vi "Read.vi"(6 "Append Index":i32, 8 "error in (no error)":errorcluster, 11 "Data.TDMS":refnum<class "LV-Data.TDMS.lvclass">) -> (0 "error out":errorcluster, 1 "Notes":string, 2 "Data (Dictionary)":T1[](array[typedef]), 3 "Data.TDMS out":refnum<class "LV-Data.TDMS.lvclass">, 5 "Path out":path)   [LabVIEW 2019, in "LV-Data.TDMS.lvclass"]
uses:
  LV-Data.TDMS.lvclass
  C:/Users/patrick/Documents/GitHub/LV-Data/src/LV-Data/LV-Data.lvclass
  LV-Data/Typedefs/Dictionary--cluster.ctl
  LV-Data.TDMS.lvclass/LV-Data.TDMS.ctl
  LV-Data/Typedefs/Operation--enum.ctl
  LV-Data/LV-Data.lvclass/LV-Data.ctl
  LV-Data/LV-Data.lvclass
  LV-Data/Typedefs/Map Variant--map.ctl
  <vilib>/Utility/miscctls.llb/LVMapReplaceAction.ctl
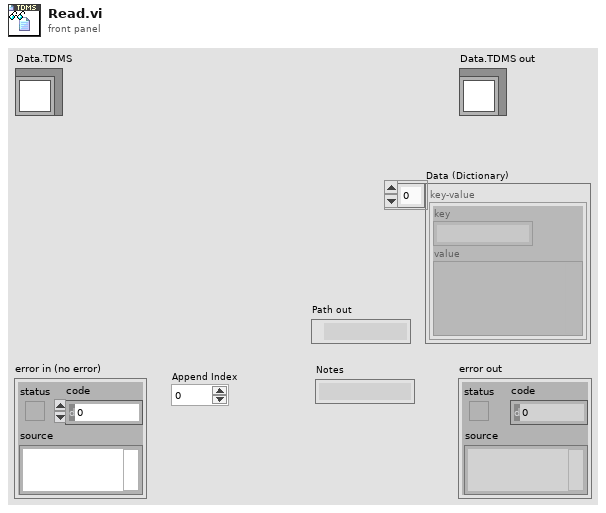
[diagram p1: front panel]
types:
  T1 = typedef "LV-Data.lvclass/Dictionary--cluster.ctl" = cluster{"key":string, "value":variant}
  T2 = typedef "LV-Data.lvclass/Operation--enum.ctl" = enum16{"Read", "Write", "Write + Append"}
  T3 = typedef "LV-Data.lvclass/Map Variant--map.ctl" = map{string, variant}
  T4 = typedef "LVMapReplaceAction.ctl" = enum32{"Modify Entry only if found", "Add or Modify Entry", "Delete Entry"}
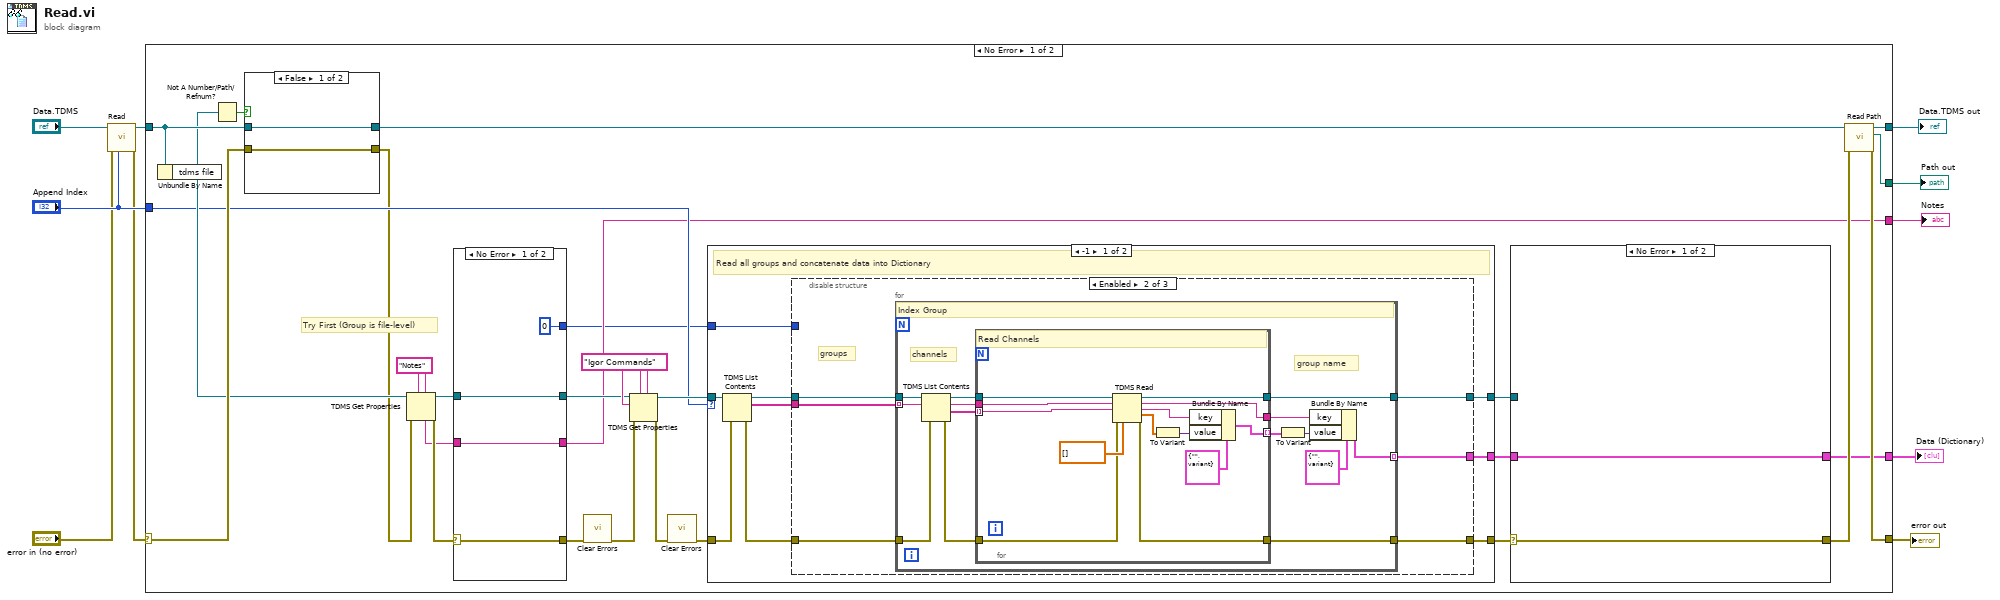
[diagram p0: block diagram]
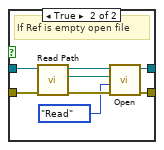
[diagram p2: hidden frame]
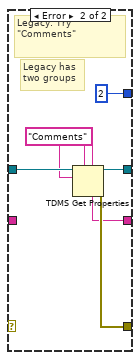
[diagram p3: hidden frame]
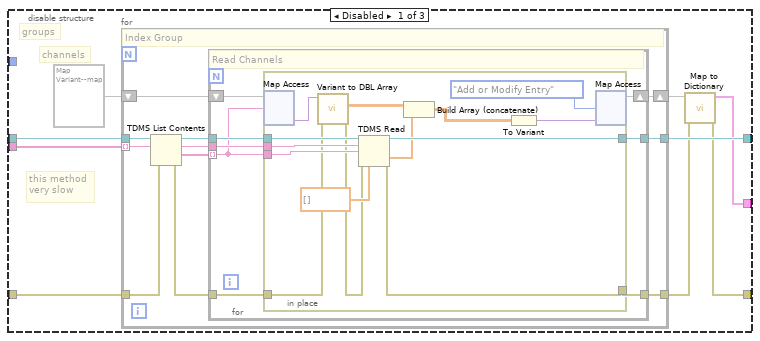
[diagram p4: hidden frame]
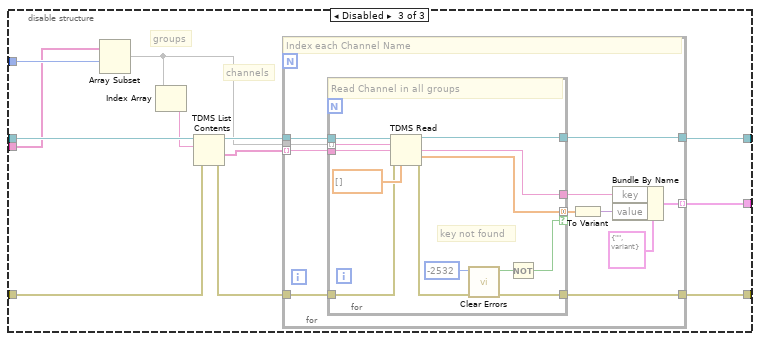
[diagram p5: hidden frame]
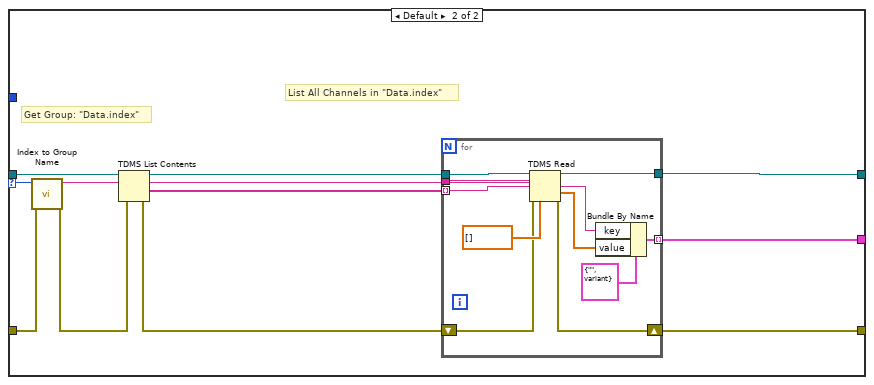
[diagram p6: hidden frame]
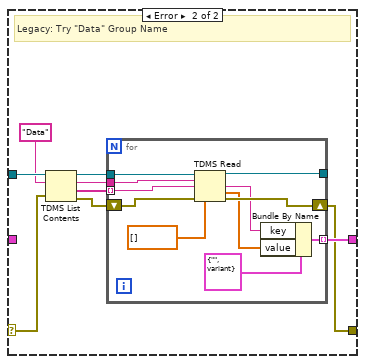
[diagram p7: hidden frame]
diagram:
  n1 = call-parent "Read.vi"("Append Index"="Append Index", "error in (no error)"="error in (no error)", "Data Save in"="Data.TDMS") -> ("error out"=w1:errorcluster, "Data Save out"=w4:refnum<class "LV-Data.TDMS.lvclass">)  [unwired: 4 in, 3 out]
  n2 = case shown="No Error" w1 {
    selector: w1 -> [w31 w223]
    tunnel: w4 -> [w33 w222]
    tunnel: [w36 w222] -> w10
    tunnel: [w35 w223] -> w9
    tunnel: [w37 _] -> w8
    tunnel: "Append Index" -> [w23 _]
    tunnel: [w13 _] -> w7
    tunnel: [w20 _] -> w6
    frame No Error {
      w27 = "Notes" ("group name")
      w30 = "Igor Commands" ("attrib name")
      # "Try First (Group is file-level)"
      n3 = Unbundle By Name(w33) -> ("tdms file"=w25:refnum<k34>)
      n4 = Not A Number/Path/Refnum?(number/path/refnum=w25) -> (NaN/Path/Refnum?=w34:bool)
      n5 = case shown="False" w34 {
        tunnel: w33 -> [w39 w47]
        tunnel: [w39 w48] -> w32
        tunnel: [w40 w44] -> w18
        tunnel: w31 -> [w40 w43]
        frame False {
        }
        frame True {
          # "If Ref is empty open file"
          n6 = call "Read Path.vi"("error in (no error)"=w43, "Data Save"=w47) -> ("error out"=w46:errorcluster, "Path"=w41:path, "Data Save out"=w45:refnum<class "LV-Data.TDMS.lvclass">)  [unwired: 7 in]
          n7 = call-dynamic "Open.vi"("error in (no error)"=w46, "Operation"=Operation--enum."Read", "Path"=w41, "Data.TDMS in"=w45) -> ("error out"=w44:errorcluster, "Data.TDMS out"=w48:refnum<class "LV-Data.TDMS.lvclass">)  [unwired: 6 in]
        }
      }
      n8 = TDMS Get Properties(5:w27, 7:w27, 8:w18, 11:w25) -> (0:w29:errorcluster, 3:w26:refnum<k34>, 4:w28:string)  [unwired: 2 in, 3 out]
      n9 = case shown="No Error" w29 {
        selector: w29 -> [w52 _]
        tunnel: [w52 w58] -> w17
        tunnel: w28 -> [w51 _]
        tunnel: [w51 w57] -> w13
        tunnel: w26 -> [w50 w56]
        tunnel: [w50 w55] -> w24
        tunnel: [0 ("index") 2 ("index")] -> w12
        frame No Error {
        }
        frame Error {
          w54 = "Comments" ("group name")
          # "Legacy has\ntwo groups"
          # "Legacy: Try \"Comments\""
          n10 = TDMS Get Properties(5:w54, 7:w54, 10:w54, 11:w56) -> (0:w58:errorcluster, 3:w55:refnum<k34>, 4:w57:string)  [unwired: 2 in, 3 out]
        }
      }
      n11 = call <vilib>:"Clear Errors.vi"("error in (no error)"=w17) -> ("error out"=w16:errorcluster)  [unwired: 5 in, 1 out]
      n12 = TDMS Get Properties(5:w30, 7:w30, 8:w16, 10:w30, 11:w24) -> (0:w15:errorcluster, 3:w38:refnum<k34>)  [unwired: 1 in, 4 out]
      n13 = call <vilib>:"Clear Errors.vi"("error in (no error)"=w15) -> ("error out"=w14:errorcluster)  [unwired: 5 in, 1 out]
      n14 = case shown="-1" w23 {
        selector: w23 -> [_ w185]
        tunnel: w38 -> [w66 w190]
        tunnel: w14 -> [w63 w184]
        tunnel: [w67 w186] -> w22
        tunnel: [w62 w182] -> w19
        tunnel: w12 -> [w61 _]
        tunnel: [w59 w179] -> w11
        frame -1 {
          # "Read all groups and concatenate data into Dictionary"
          n15 = TDMS List Contents(4:w63, 7:w66) -> (0:w64:errorcluster, 2:w60:string[], 3:w65:refnum<k34>)  [unwired: 1 in, 1 out]
          n16 = disable-structure shown="Enabled" {
            disable-tunnel: [w68 w110 w154] -> w67
            disable-tunnel: w65 -> [w74 w113 w153]
            disable-tunnel: w64 -> [w75 w114 w150]
            disable-tunnel: [w76 w115 w147] -> w62
            disable-tunnel: w61 -> [_ _ w146]
            disable-tunnel: w60 -> [w73 w112 w145]
            disable-tunnel: [w70 w111 w143] -> w59
            frame Disabled {
              # "this method\nvery slow"
              # "groups"
              # "channels"
              n17 = for {
                tunnel: [w86] -> w76
                tunnel: [w87] -> w69
                tunnel: w75 -> [w85]
                tunnel: w74 -> [w83]
                tunnel: w73 -> [w81] mode=indexing
                shift-right: [w77] -> w71
                shift-left: T3 {} ("map in") -> [w78]
                # "Index Group"
                n18 = TDMS List Contents(4:w85, 6:w81, 7:w83) -> (0:w84:errorcluster, 1:w79:string[], 2:w80:string, 3:w82:refnum<k34>)
                n19 = for {
                  tunnel: w80 -> [w94]
                  tunnel: w82 -> [w95]
                  tunnel: [w93] -> w86
                  tunnel: w84 -> [w92]
                  tunnel: [w91] -> w87
                  tunnel: w79 -> [w89] mode=indexing
                  shift-right: [w88] -> w77
                  shift-left: w78 -> [w90]
                  # "Read Channels"
                  n20 = in-place {
                    in-place-border: w95 -> [w109]
                    in-place-border: w94 -> [w108]
                    in-place-border: [w106] -> w93
                    in-place-border: w92 -> [w96]
                    in-place-border: [w105] -> w91
                    in-place-border: w89 -> [w104]
                    n21 = in-place-map #1(w90, w89) -> (w100:variant)  [unwired: 1 in, 1 out]
                    n22 = call "Variant to DBL Array.vi"("error in (no error)"=w96, "Data (Variant)"=w100) -> ("error out"=w97:errorcluster, "2D Array"=w101:dbl[][])  [unwired: 7 in, 1 out]
                    n23 = TDMS Read(0:w109, 5:w108, 7:w104, 11:w97, 12:dbl[] [] ("array type (2D Dbl)")) -> (4:w106:refnum<k34>, 10:w102:dbl[], 15:w105:errorcluster)  [unwired: 3 in, 3 out]
                    n24 = Build Array (concatenate)(w101, w102) -> (w99:dbl[][])
                    n25 = To Variant(anything=w99) -> (Variant=w98:variant)
                    n26 = in-place-map #1(w98, LVMapReplaceAction."Add or Modify Entry" ("action")) -> (w88:T3)  [unwired: 2 out]
                  }
                }
              }
              n27 = call "Map to Dictionary.vi"("error in (no error)"=w69, "map"=w71) -> ("error out"=w68:errorcluster, "Data (Dictionary)"=w70:T1[])  [unwired: 8 in]
            }
            frame Enabled {
              # "groups"
              n28 = for {
                tunnel: [w128] -> w115
                tunnel: [w129] -> w110
                tunnel: w114 -> [w127]
                tunnel: w113 -> [w125]
                tunnel: w112 -> [w123] mode=indexing
                tunnel: [w116] -> w111 mode=indexing
                # "group name"
                # "channels"
                # "Index Group"
                n29 = TDMS List Contents(4:w127, 6:w123, 7:w125) -> (0:w126:errorcluster, 1:w121:string[], 2:w122:string, 3:w124:refnum<k34>)
                n30 = for {
                  tunnel: w122 -> [w141]
                  tunnel: w124 -> [w142]
                  tunnel: [w140] -> w128
                  tunnel: w126 -> [w136]
                  tunnel: [w139] -> w129
                  tunnel: w121 -> [w138] mode=indexing
                  tunnel: [w132] -> w119 mode=indexing
                  tunnel: [w130] -> w117
                  # "Read Channels"
                  n31 = TDMS Read(0:w142, 5:w141, 7:w138, 11:w136, 12:dbl[] [] ("array type (2D Dbl)")) -> (4:w140:refnum<k34>, 6:w130:string, 8:w131:string, 10:w135:dbl[], 15:w139:errorcluster)  [unwired: 3 in, 1 out]
                  n32 = To Variant(anything=w135) -> (Variant=w133:variant)
                  n33 = Bundle By Name(cluster=T1 {"key"="", "value"=variant} ("key-value"), "key"=w131, "value"=w133) -> (w132:T1)
                }
                n34 = To Variant(anything=w119) -> (Variant=w118:variant)
                n35 = Bundle By Name(cluster=T1 {"key"="", "value"=variant} ("key-value"), "key"=w117, "value"=w118) -> (w116:T1)
              }
            }
            frame Disabled {
              # "groups"
              # "channels"
              n36 = Array Subset(array=w145, index=w146) -> (w148:string[])  [unwired: 1 in]
              n37 = Index Array(array=w148) -> (element=w149:string)  [unwired: 1 in]
              n38 = TDMS List Contents(4:w150, 6:w149, 7:w153) -> (0:w144:errorcluster, 1:w152:string[], 3:w151:refnum<k34>)  [unwired: 1 out]
              n39 = for {
                tunnel: [w158] -> w143 mode=indexing
                tunnel: w151 -> [w164]
                tunnel: w148 -> [w163]
                tunnel: w152 -> [w162] mode=indexing
                tunnel: [w156] -> w147
                tunnel: w144 -> [w157]
                tunnel: [w165] -> w154
                # "Index each Channel Name"
                n40 = for {
                  tunnel: w162 -> [w176]
                  tunnel: w163 -> [w177] mode=indexing
                  tunnel: w164 -> [w178]
                  tunnel: [w174] -> w161 mode=concatenating if=w167
                  tunnel: [w173] -> w160
                  tunnel: [w172] -> w156
                  tunnel: w157 -> [w171]
                  tunnel: [w168] -> w165
                  # "key not found"
                  # "Read Channel in all groups"
                  n41 = TDMS Read(0:w178, 5:w177, 7:w176, 11:w171, 12:dbl[] [] ("array type (2D Dbl)")) -> (4:w172:refnum<k34>, 8:w173:string, 10:w174:dbl[], 15:w169:errorcluster)  [unwired: 3 in, 2 out]
                  n42 = call <vilib>:"Clear Errors.vi"("error in (no error)"=w169, "specific error code to clear (0: all)"=-2532) -> ("error out"=w168:errorcluster, "specific error cleared?"=w166:bool)  [unwired: 4 in]
                  n43 = Not(x=w166) -> (.not. x?=w167:bool)
                }
                n44 = To Variant(anything=w161) -> (Variant=w155:variant)
                n45 = Bundle By Name(cluster=T1 {"key"="", "value"=variant} ("key-value"), "key"=w160, "value"=w155) -> (w158:T1)
              }
            }
          }
        }
        frame Default {
          # "List All Channels in \"Data.index\""
          # "Get Group: \"Data.index\""
          n46 = call "Index to Group Name.vi"("error in (no error)"=w184, "Append Index"=w185) -> ("error out"=w180:errorcluster, "group name in (Untitled)"=w183:string)  [unwired: 8 in]
          n47 = TDMS List Contents(4:w180, 6:w183, 7:w190) -> (0:w181:errorcluster, 1:w187:string[], 2:w188:string, 3:w189:refnum<k34>)
          n48 = for {
            shift-right: [w191] -> w186
            shift-left: w181 -> [w192]
            tunnel: w187 -> [w193] mode=indexing
            tunnel: w188 -> [w199]
            tunnel: [w198] -> w179 mode=indexing
            tunnel: w189 -> [w200]
            tunnel: [w194] -> w182
            n49 = TDMS Read(0:w200, 5:w199, 7:w193, 11:w192, 12:dbl[] [] ("array type (2D Dbl)")) -> (4:w194:refnum<k34>, 10:w195:dbl[], 15:w191:errorcluster)  [unwired: 3 in, 3 out]
            n50 = Bundle By Name(cluster=T1 {"key"="", "value"=variant} ("key-value"), "key"=w193, "value"=w195) -> (w198:T1)
          }
        }
      }
      n51 = case shown="No Error" w22 {
        selector: w22 -> [w201 w206]
        tunnel: [w201 w203] -> w21
        tunnel: [w202 w204] -> w20
        tunnel: w19 -> [_ w207]
        tunnel: w11 -> [w202 _]
        frame No Error {
        }
        frame Error {
          # "Legacy: Try \"Data\" Group Name"
          n52 = TDMS List Contents(4:w206, 6:"Data" ("group name"), 7:w207) -> (0:w209:errorcluster, 1:w211:string[], 2:w210:string, 3:w208:refnum<k34>)
          n53 = for {
            shift-right: [w219] -> w203
            shift-left: w209 -> [w221]
            tunnel: w211 -> [w212] mode=indexing
            tunnel: w210 -> [w218]
            tunnel: [w217] -> w204 mode=indexing
            tunnel: w208 -> [w220]
            tunnel: [w213] -> _
            n54 = TDMS Read(0:w220, 5:w218, 7:w212, 11:w221, 12:dbl[] [] ("array type (2D Dbl)")) -> (4:w213:refnum<k34>, 10:w214:dbl[], 15:w219:errorcluster)  [unwired: 3 in, 3 out]
            n55 = Bundle By Name(cluster=T1 {"key"="", "value"=variant} ("key-value"), "key"=w212, "value"=w214) -> (w217:T1)
          }
        }
      }
      n56 = call "Read Path.vi"("error in (no error)"=w21, "Data Save"=w32) -> ("error out"=w35:errorcluster, "Path"=w37:path, "Data Save out"=w36:refnum<class "LV-Data.TDMS.lvclass">)  [unwired: 7 in]
    }
    frame Error {
    }
  }
  "error out" <- w9
  "Data.TDMS out" <- w10
  "Path out" <- w8
  "Data (Dictionary)" <- w6
  "Notes" <- w7
